vi "Disabled.vi"(7 "Robot Mode":T2, 10 "Match Info":T1={"Autonomous Elapsed Seconds"=0.0, "TeleOp Elapsed Seconds"=0.0, "Disabled Elapsed Seconds"=0.0, "Visited Autonomous"=FALSE, "Visited TeleOp"=FALSE, "Visited Disabled"=FALSE, "Autonomous Settings"={"Autonomous Style"=enum."Independent", "VI Refnum"=refnum}}, 11 "Call Context":T3) -> ()   [LabVIEW 2012]
doc: "This VI is called each time a disabled packet is received from the DS. It is often used to prepare for the next robot mode, to calibrate sensors, etc."
uses:
  <vilib>/Rock Robotics/WPI/DriverStation/WPI_DriverStationDerivedRobotMode.ctl
  <vilib>/Rock Robotics/WPI/DriverStation/WPI_DriverStationRobotMode2.ctl
  <vilib>/Rock Robotics/WPI/DriverStation/WPI_DriverStationMatch Info.ctl
  Robot Global Data.vi
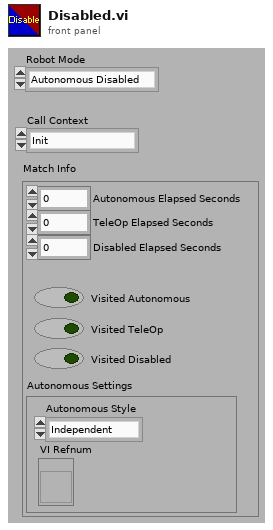
[diagram p1: front panel]
types:
  T1 = typedef "WPI_DriverStationMatch Info.ctl" = cluster{"Autonomous Elapsed Seconds":dbl, "TeleOp Elapsed Seconds":dbl, "Disabled Elapsed Seconds":dbl, "Visited Autonomous":bool, "Visited TeleOp":bool, "Visited Disabled":bool, "Autonomous Settings":cluster{"Autonomous Style":enum16{"Iterative", "Independent"}, "VI Refnum":refnum<vi>}}
  T2 = typedef "WPI_DriverStationRobotMode2.ctl" = enum16{"Autonomous Disabled", "Autonomous Enabled", "Teleop Disabled", "Teleop Enabled", "Timeout", "Finish", "Test Disabled", "Test Enabled"}
  T3 = typedef "WPI_DriverStationDerivedRobotMode.ctl" = enum16{"Init", "Execute", "Stop"}
  T4 = typedef "WPI_MotorControlDeviceRef.ctl" = cluster{"DeviceStatus":errorcluster, "Type":enum16{"PWM", "CAN"}, "PWM":cluster{"Digital Module":T5, "PWM Channel":T6, "DeadBand":T7}, "CAN":cluster{"Device Number":u8, "Control Mode":T8, "Semaphore":T9, "Max Vout":dbl}, "Invert":bool, "TransformRef":T10, "InvTransformRef":T10}
  T5 = typedef "FPGA_TypedefDigitalModule.ctl" = enum16{"Digital Module 1", "Digital Module 2"}
  T6 = typedef "FPGA_DIOPWMChannel.ctl" = enum8{"PWM 1", "PWM 2", "PWM 3", "PWM 4", "PWM 5", "PWM 6", "PWM 7", "PWM 8", "PWM 9", "PWM 10", "Invalid"}
  T7 = typedef "WPI_PWMDeadband.ctl" = cluster{"Name":string, "maxPositivePwm":i32, "minPositivePwm":i32, "centerPwm":i32, "maxNegativePwm":i32, "minNegativePwm":i32, "angularRange":u16}
  T8 = typedef "WPI_CANJaguar_ControlMode.ctl" = enum8{"Percent VBus", "Current", "Speed", "Position", "Voltage"}
  T9 = typedef "Semaphore RefNum" = refnum<k1>
  T10 = typedef "WPI_PWMTransform_ConPane.ctl" = refnum<vi>
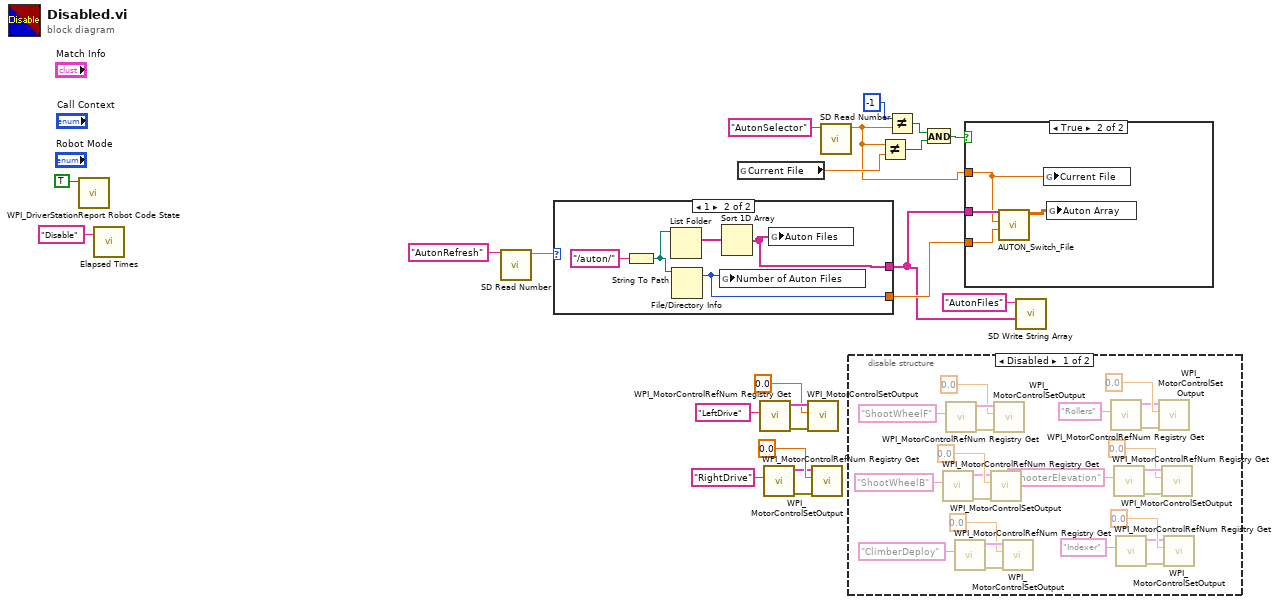
[diagram p0: block diagram]
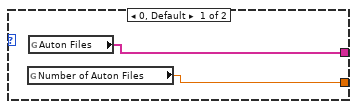
[diagram p4: hidden frame]
diagram:
  n1 = call <vilib>:"WPI_DriverStationReport Robot Code State.vi"("Disabled"=TRUE ("Autonomous")) -> ()  [unwired: 10 in, 1 out]
  n2 = call "Elapsed Times.vi"("Call Name"="Disable") -> ()  [unwired: 2 in, 1 out]
  n3 = call <vilib>:"SD Read Number.vi"("Name"="AutonRefresh") -> ("Numeric"=w2:dbl)  [unwired: 8 in, 2 out]
  n4 = case shown="1" w2 {
    tunnel: [w23 w26] -> w12
    tunnel: [w24 w25] -> w7
    frame 0, Default {
      n5 = global read "Robot Global Data.vi" "Number of Auton Files"() -> (w23:dbl)
      n6 = global read "Robot Global Data.vi" "Auton Files"() -> (w24:string[])
    }
    frame 1 {
      n7 = String To Path(string="/auton/") -> (path=w28:path)
      n8 = List Folder(path=w28) -> (filenames=w27:string[])  [unwired: 3 in, 3 out]
      n9 = File/Directory Info(path=w28) -> (size=w26:i64)  [unwired: 1 in, 6 out]
      n10 = global write "Robot Global Data.vi" "Number of Auton Files"(w26) -> ()
      n11 = Sort 1D Array(array=w27) -> (sorted array=w25:string[])
      n12 = global write "Robot Global Data.vi" "Auton Files"(w25) -> ()
    }
  }
  n13 = global read "Robot Global Data.vi" "Current File"() -> (w10:dbl)
  n14 = call <vilib>:"WPI_MotorControlRefNum Registry Get.vi"("refnum name"="LeftDrive") -> ("error out"=w20:errorcluster, "MotorControlDevRef"=w19:T4)  [unwired: 9 in]
  n15 = call <vilib>:"WPI_MotorControlRefNum Registry Get.vi"("refnum name"="RightDrive") -> ("error out"=w13:errorcluster, "MotorControlDevRef"=w14:T4)  [unwired: 9 in]
  n16 = call <vilib>:"WPI_MotorControlSetOutput.vi"("error in (no error)"=w20, "Output"=0.0, "MotorControlDevRef"=w19) -> ()  [unwired: 6 in, 3 out]
  n17 = call <vilib>:"WPI_MotorControlSetOutput.vi"("error in (no error)"=w13, "Output"=0.0, "MotorControlDevRef"=w14) -> ()  [unwired: 6 in, 3 out]
  n18 = call <vilib>:"SD Read Number.vi"("Name"="AutonSelector") -> ("Numeric"=w3:dbl)  [unwired: 8 in, 2 out]
  n19 = disable-structure shown="Disabled" {
    frame Disabled {
      n20 = call <vilib>:"WPI_MotorControlRefNum Registry Get.vi"("refnum name"="ShootWheelB") -> ("error out"=w46:errorcluster, "MotorControlDevRef"=w47:T4)  [unwired: 9 in]
      n21 = call <vilib>:"WPI_MotorControlRefNum Registry Get.vi"("refnum name"="ShootWheelF") -> ("error out"=w53:errorcluster, "MotorControlDevRef"=w52:T4)  [unwired: 9 in]
      n22 = call <vilib>:"WPI_MotorControlRefNum Registry Get.vi"("refnum name"="ClimberDeploy") -> ("error out"=w45:errorcluster, "MotorControlDevRef"=w44:T4)  [unwired: 9 in]
      n23 = call <vilib>:"WPI_MotorControlSetOutput.vi"("error in (no error)"=w46, "Output"=0.0, "MotorControlDevRef"=w47) -> ()  [unwired: 6 in, 3 out]
      n24 = call <vilib>:"WPI_MotorControlSetOutput.vi"("error in (no error)"=w53, "Output"=0.0, "MotorControlDevRef"=w52) -> ()  [unwired: 6 in, 3 out]
      n25 = call <vilib>:"WPI_MotorControlSetOutput.vi"("error in (no error)"=w45, "Output"=0.0, "MotorControlDevRef"=w44) -> ()  [unwired: 6 in, 3 out]
      n26 = call <vilib>:"WPI_MotorControlRefNum Registry Get.vi"("refnum name"="Rollers") -> ("error out"=w38:errorcluster, "MotorControlDevRef"=w39:T4)  [unwired: 9 in]
      n27 = call <vilib>:"WPI_MotorControlRefNum Registry Get.vi"("refnum name"="ShooterElevation") -> ("error out"=w37:errorcluster, "MotorControlDevRef"=w36:T4)  [unwired: 9 in]
      n28 = call <vilib>:"WPI_MotorControlRefNum Registry Get.vi"("refnum name"="Indexer") -> ("error out"=w30:errorcluster, "MotorControlDevRef"=w31:T4)  [unwired: 9 in]
      n29 = call <vilib>:"WPI_MotorControlSetOutput.vi"("error in (no error)"=w38, "Output"=0.0, "MotorControlDevRef"=w39) -> ()  [unwired: 6 in, 3 out]
      n30 = call <vilib>:"WPI_MotorControlSetOutput.vi"("error in (no error)"=w37, "Output"=0.0, "MotorControlDevRef"=w36) -> ()  [unwired: 6 in, 3 out]
      n31 = call <vilib>:"WPI_MotorControlSetOutput.vi"("error in (no error)"=w30, "Output"=0.0, "MotorControlDevRef"=w31) -> ()  [unwired: 6 in, 3 out]
    }
    frame Enabled {
    }
  }
  n32 = Not Equal?(x=w3, y=w10) -> (x != y?=w8:bool)
  n33 = Not Equal?(x=-1, y=w3) -> (x != y?=w9:bool)
  n34 = And(x=w9, y=w8) -> (x .and. y?=w5:bool)
  n35 = case shown="True" w5 {
    tunnel: w7 -> [_ w57]
    tunnel: w12 -> [_ w56]
    tunnel: w3 -> [_ w54]
    frame False {
    }
    frame True {
      n36 = call "AUTON_Switch_File.vi"("Number of Auton Files"=w56, "Auton File"=w54, "Auton Files"=w57) -> ("Auton Array"=w55:dbl[][])  [unwired: 7 in, 1 out]
      n37 = global write "Robot Global Data.vi" "Current File"(w54) -> ()
      n38 = global write "Robot Global Data.vi" "Auton Array"(w55) -> ()
    }
  }
  n39 = call <vilib>:"SD Write String Array.vi"("String Array"=w7, "Name"="AutonFiles") -> ()  [unwired: 8 in, 2 out]
